vi "Servo PWM FPGA.vi"() -> ()   [LabVIEW 2015]
uses:
  <vilib>/rvi/Emulation/niFpgaGetClockAttributes.vi
  <vilib>/rvi/Emulation/niFpgaSctlEmulationGetInTimedLoop.vi
  <vilib>/rvi/Emulation/niFpgaEmulationReportErrorSimple.vi
  <vilib>/rvi/eio/common/nirviEmuTemplateMethod_errors.vi
  <vilib>/rvi/Emulation/niFpgaCriticalErrorInLSC.vi
  <vilib>/eio/EIONode/EIONode.xnode
panel:
  in  "SERVO Y":i16
  in  "SERVO X":i16
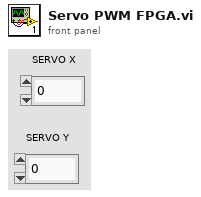
[diagram p1: front panel]
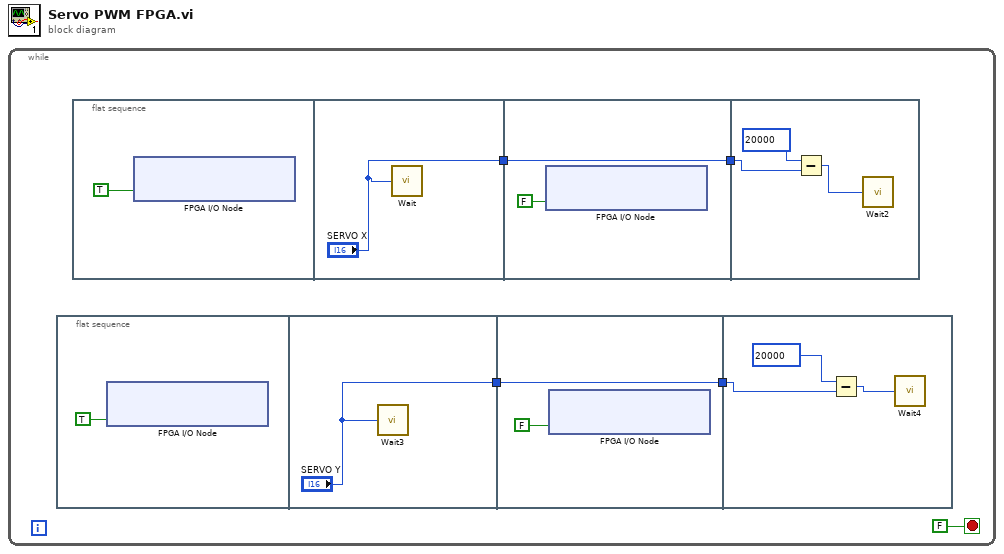
[diagram p0: block diagram]
diagram:
  n1 = while {
    stop <- FALSE stop-if-true
    n2 = flat-sequence {
      tunnel: ["SERVO Y"] -> w2
      tunnel: w2 -> [w8]
      tunnel: [w8] -> w1
      tunnel: w1 -> [w12]
      frame #0 {
        n3 = xnode "FPGA I/O Node"("ConnectorA/DIO9"=TRUE) -> ()  [unwired: 1 in, 1 out]
      }
      frame #1 {
        n4 = call "Wait3"("Count(uSec)"="SERVO Y") -> ()  [unwired: 1 out]
      }
      frame #2 {
        n5 = xnode "FPGA I/O Node"("ConnectorA/DIO9"=FALSE) -> ()  [unwired: 1 in, 1 out]
      }
      frame #3 {
        n6 = Subtract(x=i16 20000, y=w12) -> (x-y=w11:i16)
        n7 = call "Wait4"("Count(uSec)"=w11) -> ()  [unwired: 1 out]
      }
    }
    n8 = flat-sequence {
      tunnel: ["SERVO X"] -> w5
      tunnel: w5 -> [w15]
      tunnel: [w15] -> w4
      tunnel: w4 -> [w19]
      frame #0 {
        n9 = xnode "FPGA I/O Node"("ConnectorA/DIO8"=TRUE) -> ()  [unwired: 1 in, 1 out]
      }
      frame #1 {
        n10 = call "Wait"("Count(uSec)"="SERVO X") -> ()  [unwired: 1 out]
      }
      frame #2 {
        n11 = xnode "FPGA I/O Node"("ConnectorA/DIO8"=FALSE) -> ()  [unwired: 1 in, 1 out]
      }
      frame #3 {
        n12 = Subtract(x=u32 20000, y=w19) -> (x-y=w17:u32)
        n13 = call "Wait2"("Count(uSec)"=w17) -> ()  [unwired: 1 out]
      }
    }
  }
